vi "Query Protections.vi"(7 "Slave Address":i32=-1 min=-1 max=30 step=1, 8 "error":errorcluster, 11 "VISA":refnum<visa-resource-name>) -> (0 "error out":errorcluster, 1 "UVL":dbl format="%.3f", 2 "OVP":dbl format="%.3f", 3 "VISA out":refnum<visa-resource-name>, 4 "FB":bool)   [LabVIEW 2025, in "TDK-Lambda GEN LAN Series.lvlib"]
doc: "Queries the GEN and returns:\n- Under-Voltage Limit (UVL) setting in volts\n- Over-Voltage Level (OVP) setting in volts\n- Fold-Back Protection (FB) enabled as True or False"
uses:
  <userlib>/TDK-Lambda GEN LAN Series/TDK-Lambda GEN LAN Series.lvlib
panel:
  # "Read Protections:\n    Under-Voltage Limit    (UVL)\n    Over-Voltage Level     (OVP)\n    Fold-Back Enabled       (FB)"
  # "TDK-Lambda Genesys \n LAN\n  DC Power Supplies"
  # "(c) 2019 TDK-Lambda.  ALL RIGHTS RESERVED."
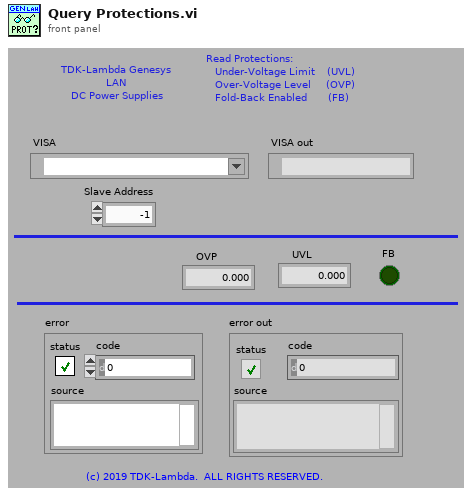
[diagram p1: front panel]
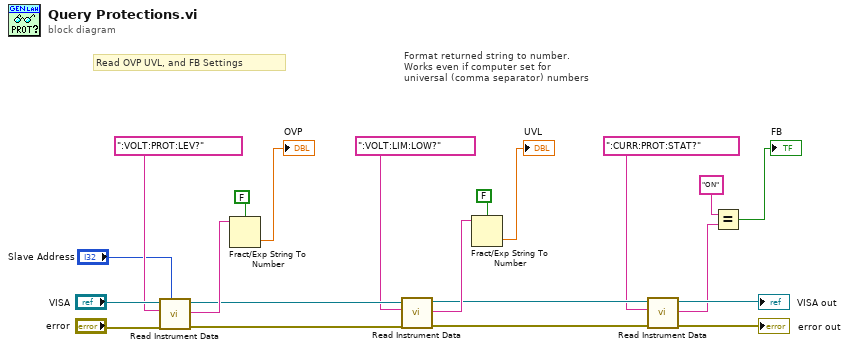
[diagram p0: block diagram]
diagram:
  # "Format returned string to number.\nWorks even if computer set for \nuniversal (comma separator) numbers"
  # "Read OVP UVL, and FB Settings"
  n1 = call <userlib>:"Read Instrument Data.vi"("Slave Address"="Slave Address", "error"="error", "Query"=":VOLT:PROT:LEV?", "VISA"="VISA") -> ("error out"=w12:errorcluster, "Response"=w17:string, "VISA out"=w13:refnum<visa-resource-name>)  [unwired: 4 in, 1 out]
  n2 = Fract/Exp String To Number(use system decimal point (T)=FALSE, string=w17) -> (number=→"OVP":dbl)  [unwired: 2 in, 1 out]
  n3 = call <userlib>:"Read Instrument Data.vi"("error"=w12, "Query"=":VOLT:LIM:LOW?", "VISA"=w13) -> ("error out"=w8:errorcluster, "Response"=w15:string, "VISA out"=w9:refnum<visa-resource-name>)  [unwired: 5 in, 1 out]
  n4 = Fract/Exp String To Number(use system decimal point (T)=FALSE, string=w15) -> (number=→"UVL":dbl)  [unwired: 2 in, 1 out]
  n5 = call <userlib>:"Read Instrument Data.vi"("error"=w8, "Query"=":CURR:PROT:STAT?", "VISA"=w9) -> ("error out"=→"error out":errorcluster, "Response"=w4:string, "VISA out"=→"VISA out":refnum<visa-resource-name>)  [unwired: 5 in, 1 out]
  n6 = Equal?(x="ON", y=w4) -> (x = y?=→"FB":bool)
